vi "piezol wave.vi"(9 "position step":dbl, 10 "position offset":dbl, 11 "frame#":dbl) -> (3 "voltage":dbl[](array[numeric]))   [LabVIEW 2015]
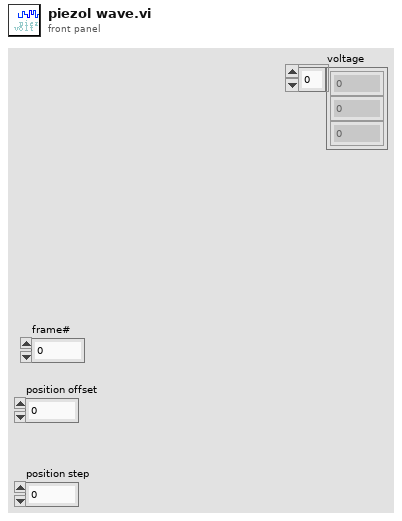
[diagram p1: front panel]
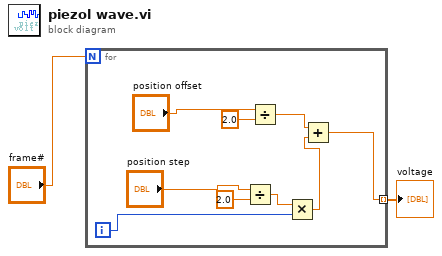
[diagram p0: block diagram]
diagram:
  n1 = for {
    N: "frame#" -> [_]
    tunnel: [w6] -> w1 mode=indexing
    i -> [w4]
    n2 = Divide(x="position step", y=2.0) -> (x/y=w5:dbl)
    n3 = Divide(x="position offset", y=2.0) -> (x/y=w7:dbl)
    n4 = Multiply(x=w5, y=w4) -> (x*y=w3:dbl)
    n5 = Add(x=w7, y=w3) -> (x+y=w6:dbl)
  }
  "voltage" <- w1
